vi "OTP - Decode Message.vi"(7 "Keys File Path":path, 11 "message (ciphered Text)":string="\"Neque porro quisquam est qui dolorem ipsum quia dolor sit amet, consectetur, adipisci velit...\"\n\"There is no one who loves pain itself, who seeks after it and wants to have it, simply because it is pain...\"") -> (3 "message (Plain Text)":string)   [LabVIEW 2013]
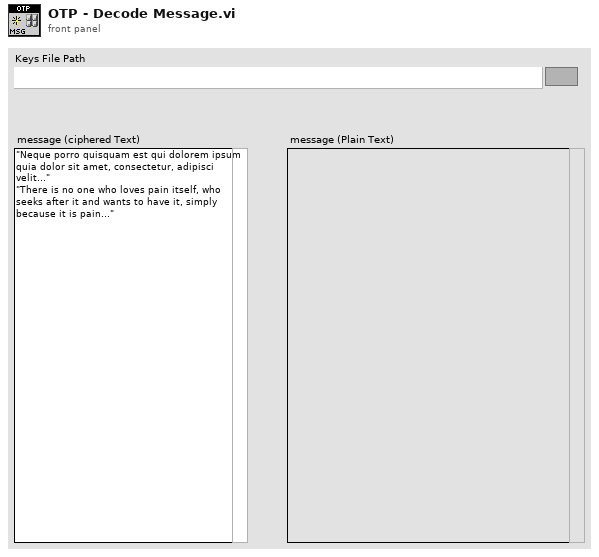
[diagram p1: front panel]
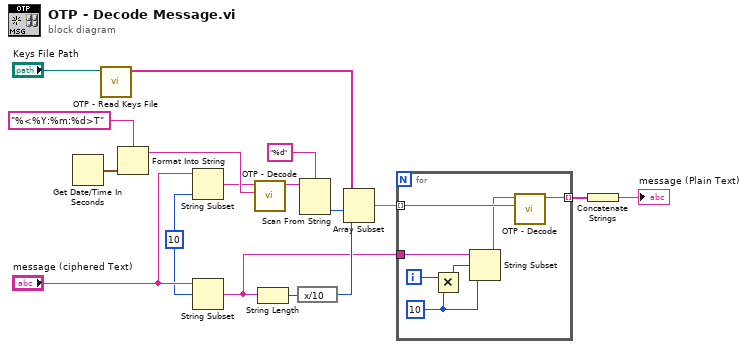
[diagram p0: block diagram]
diagram:
  w4 = 10 ("offset (0)")
  n1 = Get Date/Time In Seconds() -> (seconds since 1Jan1904=w15:timestamp)
  n2 = call "OTP - Read Keys File.vi"("File Path"="Keys File Path") -> ("keys"=w16:string[])  [unwired: 10 in]
  n3 = Format Into String(format string="%<%Y:%m:%d>T", w15) -> (resulting string=w13:string)  [unwired: 2 in, 1 out]
  n4 = String Subset(string="message (ciphered Text)", length (rest)=w4) -> (substring=w11:string)  [unwired: 1 in]
  n5 = String Subset(string="message (ciphered Text)", offset (0)=w4) -> (substring=w3:string)  [unwired: 1 in]
  n6 = call "OTP - Decode.vi"("Key (Private)"=w13, "ciphertext (Public)"=w11) -> ("original message"=w10:string)  [unwired: 9 in]
  n7 = String Length(string=w3) -> (length=w6:i32)
  n8 = expression code="x/10"(w6) -> (w5:i32)
  n9 = Scan From String(format string="%d", input string=w10) -> (output 1=w8:i32)  [unwired: 3 in, 3 out]
  n10 = Array Subset(array=w16, index=w8, length=w5) -> (w7:string[])
  n11 = for {
    tunnel: w7 -> [w20] mode=indexing
    tunnel: w3 -> [w24]
    tunnel: [w18] -> w2 mode=indexing
    i -> [w23]
    w21 = 10 ("length (rest)")
    n12 = Multiply(x=w23, y=w21) -> (x*y=w22:i32)
    n13 = String Subset(string=w24, offset (0)=w22, length (rest)=w21) -> (substring=w19:string)
    n14 = call "OTP - Decode.vi"("Key (Private)"=w20, "ciphertext (Public)"=w19) -> ("original message"=w18:string)  [unwired: 9 in]
  }
  n15 = Concatenate Strings(w2) -> (→"message (Plain Text)":string)
